vi "RemoveDrift.vi"(4 "Keep Mean?(T)":bool=TRUE, 5 "Transpose?(T)":bool=TRUE, 6 "Detrend in Polar?(F)":bool, 7 "Drift degree":dbl=3.0, 11 "Data In":cdb[][](array[numeric])=[[1.0+0.0i, 0.0+1.0i, 1.0+0.0i], [2.0+0.0i, 0.25+0.75i, 5.0+0.0i], [3.0+0.0i, 0.5+0.5i, 0.0+0.0i], [4.0+0.0i, 0.75+0.25i, 0.0+0.0i], [5.0+0.0i, 1.0+0.0i, 0.0+0.0i]] format="%#_1p") -> (3 "Data Drift Removed":cdb[][](array[numeric])=[[-2.220446049250313e-16+2.563950248511419e-16i, -5.551115123125783e-16+5.551115123125783e-16i, 2.220446049250313e-16-1.8769418499892072e-16i], [-1.3322676295501878e-15+1.2819751242557095e-16i, -2.4424906541753444e-15+4.440892098500626e-16i, 1.7763568394002505e-15-3.158916974244917e-16i], [-4.440892098500626e-16+1.2819751242557095e-16i, -8.881784197001252e-16+2.7755575615628914e-16i, 0.0-9.384709249946036e-17i], [-8.881784197001252e-16+6.409875621278547e-17i, -4.440892098500626e-16+1.3877787807814457e-16i, 0.0-4.692354624973018e-17i], [0.0+0.0i, 0.0+0.0i, 8.881784197001252e-16+0.0i]])   [LabVIEW 2021]
panel:
  out "Ang Mat":cdb[][](array[numeric]) format="%#_3p"
  out "Phase":dbl[](graph)
  out "standard deviation  pre":dbl format="%_3p"
  out "standard deviation post":dbl format="%_3p"
  in  "Harm index":i32
  out "Post-Correction":dbl[][](graph)
  out "Means Mat":cdb[][](array[numeric]) format="%#_3p"
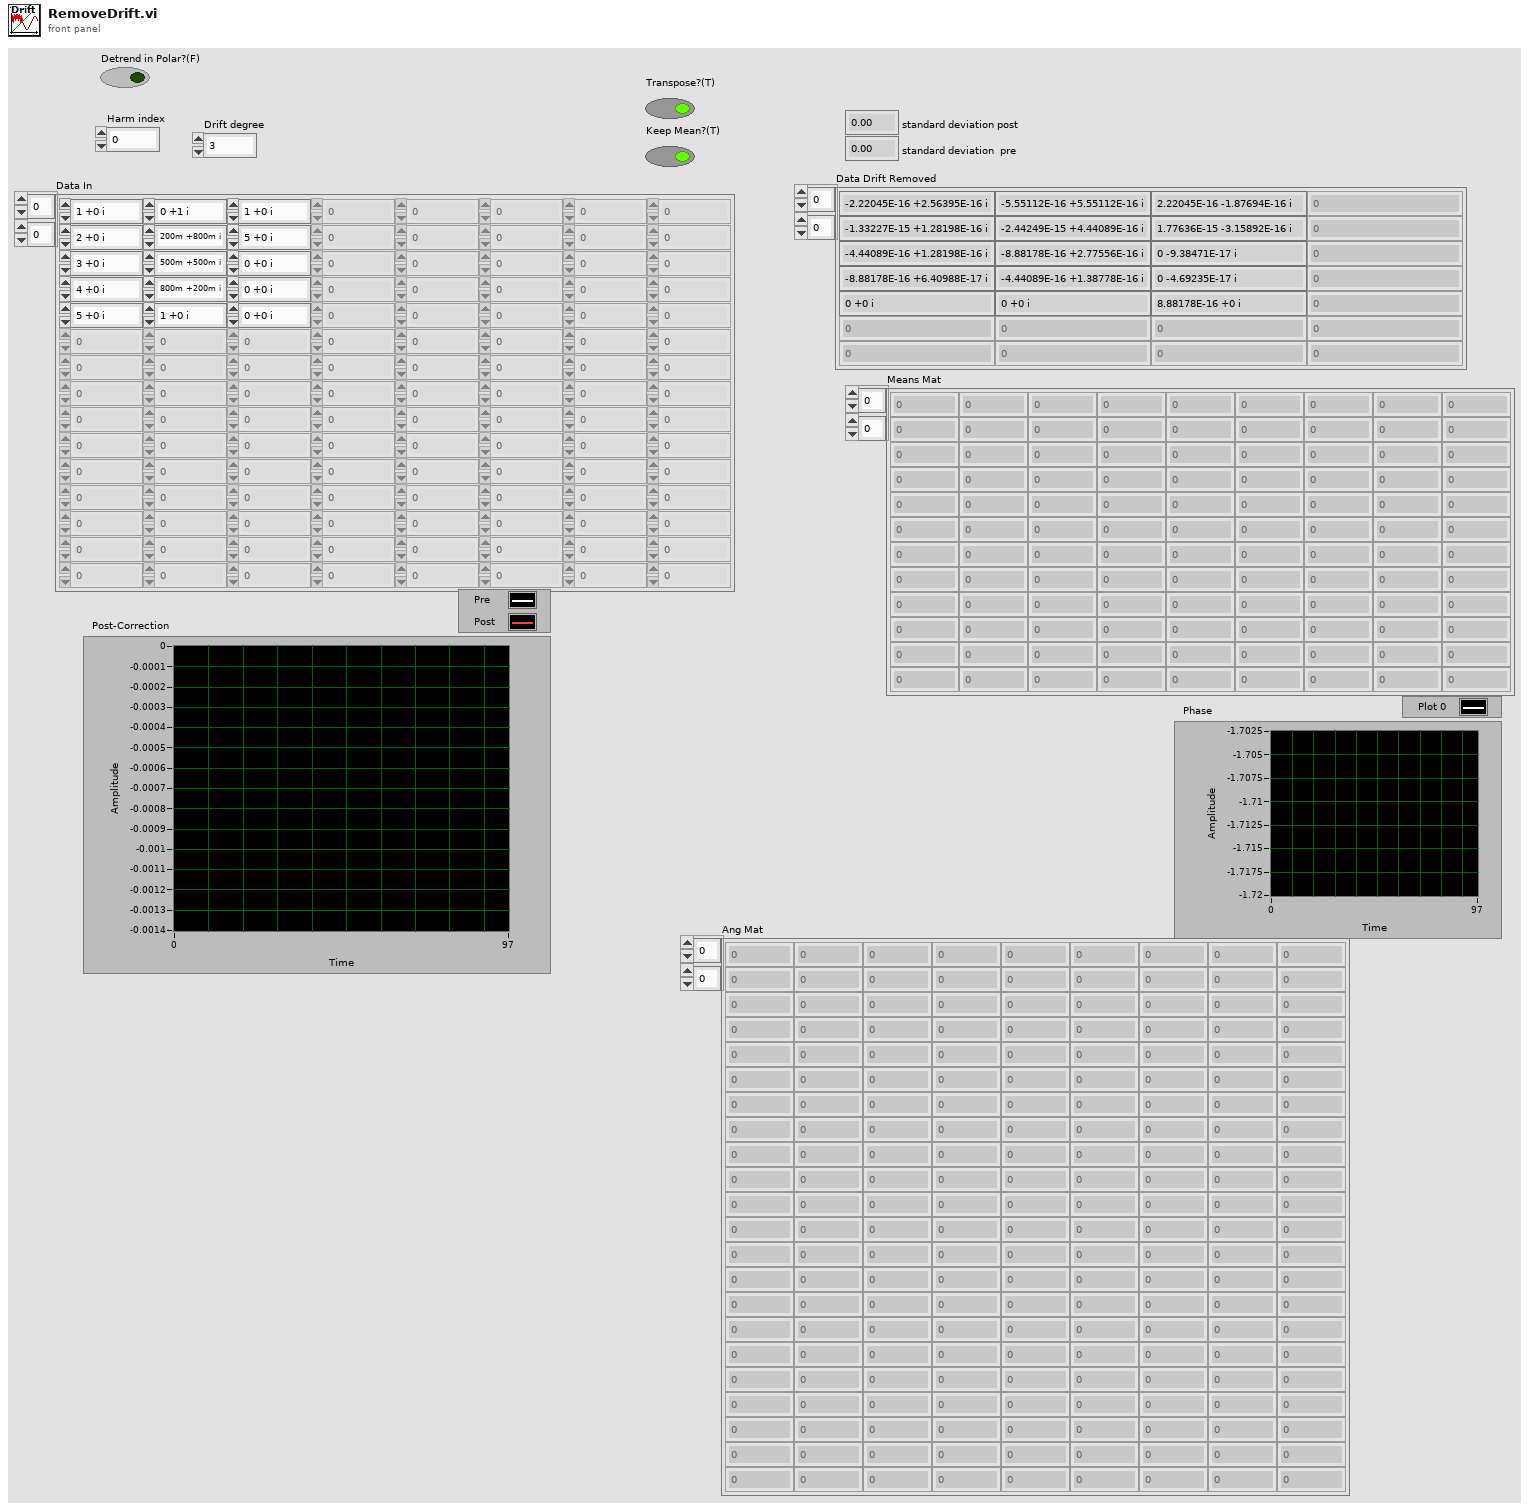
[diagram p1: front panel]
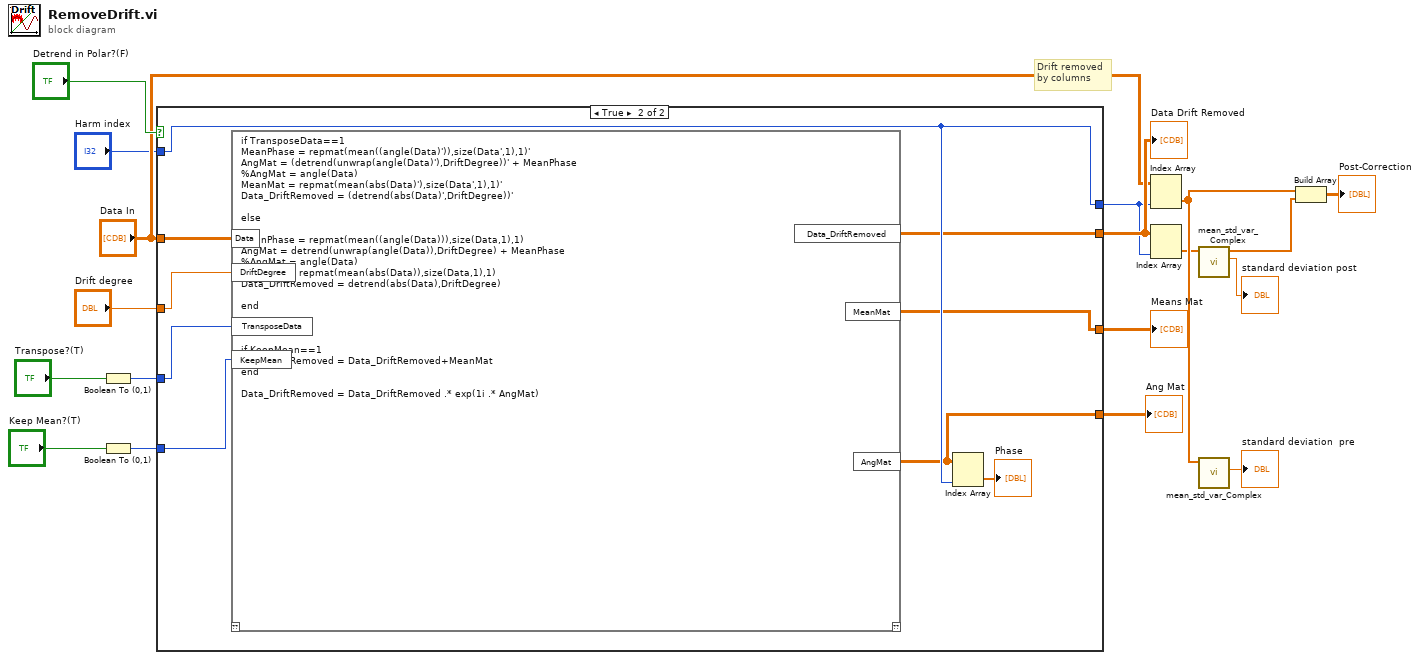
[diagram p0: block diagram]
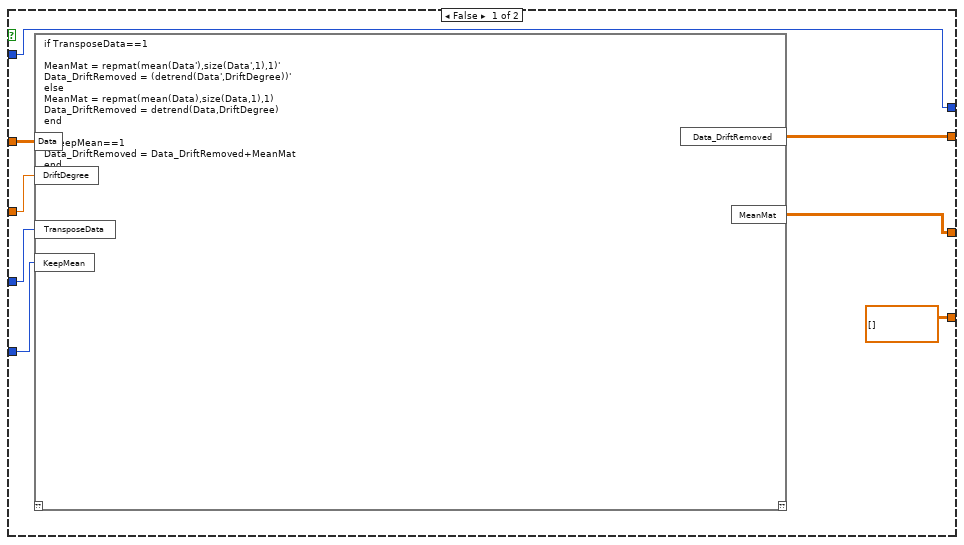
[diagram p2: hidden frame]
diagram:
  # "Drift removed\nby columns"
  n1 = Boolean To (0,1)(Boolean="Transpose?(T)") -> (0, 1=w15:i16)
  n2 = Boolean To (0,1)(Boolean="Keep Mean?(T)") -> (0, 1=w13:i16)
  n3 = case shown="True" "Detrend in Polar?(F)" {
    tunnel: [w25 w30] -> w10
    tunnel: "Data In" -> [w24 w31]
    tunnel: "Drift degree" -> [w23 w34]
    tunnel: w15 -> [w22 w33]
    tunnel: w13 -> [w21 w26]
    tunnel: [w20 w28] -> w12
    tunnel: [w19 w32] -> w8
    tunnel: "Harm index" -> [w19 w32]
    tunnel: [cdb[][] [] w27] -> w1
    frame False {
      n4 = script code="if TransposeData==1\n\nMeanMat = repmat(mean(Data'),size(Data',1),1)'\nData_DriftRemoved = (detrend(Data',DriftDegree))'\nelse\nMeanMat = repmat(mean(Data),size(Data,1),1)\nData_DriftRemoved = detrend(Data,DriftDegree)\nend\n\nif KeepMean==1\nData_DriftRemoved = Data_DriftRemoved+MeanMat\nend"("Data"=w24, "DriftDegree"=w23, "TransposeData"=w22, "KeepMean"=w21) -> ("Data_DriftRemoved"=w25:cdb[][], "MeanMat"=w20:cdb[][])  [unwired: 1 in, 1 out]
    }
    frame True {
      n5 = script code="if TransposeData==1\nMeanPhase = repmat(mean((angle(Data)')),size(Data',1),1)'\nAngMat = (detrend(unwrap(angle(Data)'),DriftDegree))' + MeanPhase\n%AngMat = angle(Data) \nMeanMat = repmat(mean(abs(Data)'),size(Data',1),1)'\nData_DriftRemoved = (detrend(abs(Data)',DriftDegree))'\n\nelse\n\nMeanPhase = repmat(mean((angle(Data))),size(Data,1),1)\nAngMat = detrend(unwrap(angle(Data)),DriftDegree) + MeanPhase\n%AngMat = angle(Data)\nMeanMat = repmat(mean(abs(Data)),size(Data,1),1)\nData_DriftRemoved = detrend(abs(Data),DriftDegree)\n\nend\n\n\n\nif KeepMean==1\nData_DriftRemoved = Data_DriftRemoved+MeanMat\nend\n\nData_DriftRemoved = Data_DriftRemoved .* exp(1i .* AngMat)"("Data"=w31, "DriftDegree"=w34, "TransposeData"=w33, "KeepMean"=w26) -> ("Data_DriftRemoved"=w30:cdb[][], "MeanMat"=w28:cdb[][], "AngMat"=w27:cdb[][])  [unwired: 1 in, 1 out]
      n6 = Index Array(array=w27, index (col)=w32) -> (element=→"Phase":cdb[])  [unwired: 1 in]
    }
  }
  "Data Drift Removed" <- w10
  "Means Mat" <- w12
  "Ang Mat" <- w1
  n7 = Index Array(array="Data In", index (col)=w8) -> (element=w3:cdb[])  [unwired: 1 in]
  n8 = Index Array(array=w10, index (col)=w8) -> (element=w2:cdb[])  [unwired: 1 in]
  n9 = call "mean_std_var_Complex.vi"("Input Array"=w2) -> ("standard deviation"=→"standard deviation post":dbl)  [unwired: 8 in, 2 out]
  n10 = call "mean_std_var_Complex.vi"("Input Array"=w3) -> ("standard deviation"=→"standard deviation  pre":dbl)  [unwired: 8 in, 2 out]
  n11 = Build Array(w3, w2) -> (→"Post-Correction":cdb[][])
